vi "SubBusFPGA.vi"(6 "1/R":fxp<+,20,0>, 9 "e3":bool, 10 "e2":bool, 11 "e1":bool) -> (2 "1-T/(RC)":fxp<+,20,0>, 3 "T/C":fxp<+,20,0>)   [LabVIEW 2015]
uses:
  <vilib>/rvi/FXPMathLib/FxpDiv/subVIs/nifxpmath_Div_SimConfig.ctl
  <vilib>/rvi/FXPMathLib/FxpDiv/simVIs/DllFxpDivTemp_sub.vi
  <vilib>/rvi/FXPMathLib/FxpAdd/XNode/nifxpmath_Add.xnode
  <vilib>/rvi/FXPMathLib/FxpDiv/XNode/nifxpmath_Div.xnode
  <vilib>/rvi/FXPMathLib/FxpMul/XNode/nifxpmath_Multiplier.xnode
  <vilib>/rvi/FXPMathLib/FxpSub/XNode/nifxpmath_Sub.xnode
  <vilib>/rvi/FXPMathLib/sim/FxpSim.dll
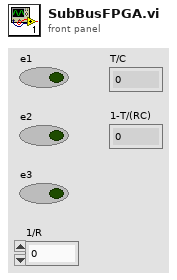
[diagram p1: front panel]
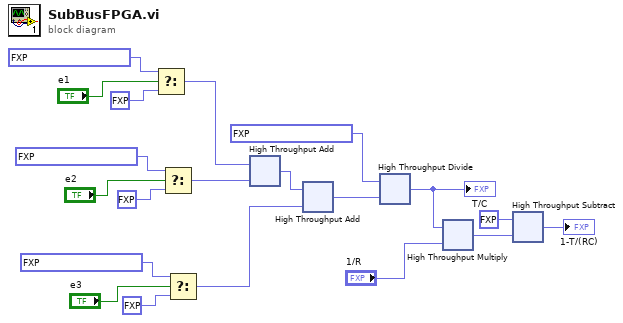
[diagram p0: block diagram]
diagram:
  n1 = Select(t=fxp<+,20,0> 4.673004150390625e-05, s="e1", f=fxp<+,20,0> 0.0) -> (s? t:f=w10:fxp<+,20,0>)
  n2 = Select(t=fxp<+,20,0> 4.673004150390625e-05, s="e2", f=fxp<+,20,0> 0.0) -> (s? t:f=w11:fxp<+,20,0>)
  n3 = Select(t=fxp<+,20,0> 4.673004150390625e-05, s="e3", f=fxp<+,20,0> 0.0) -> (s? t:f=w13:fxp<+,20,0>)
  n4 = xnode "High Throughput Add"("x"=w10, "y"=w11) -> ("x+y"=w12:fxp<+,20,0>)
  n5 = xnode "High Throughput Add"("x"=w12, "y"=w13) -> ("x+y"=w14:fxp<+,20,0>)
  n6 = xnode "High Throughput Divide"("x"=fxp<+,20,0> 1.621246337890625e-05, "y"=w14) -> ("x/y"=w17:fxp<+,20,0>)
  "T/C" <- w17
  n7 = xnode "High Throughput Multiply"("x"=w17, "y"="1/R") -> ("x*y"=w19:fxp<+,40,0>)
  n8 = xnode "High Throughput Subtract"("x"=fxp<+,1,1> 1.0, "y"=w19) -> ("x-y"=→"1-T/(RC)":fxp<+,20,0>)
